vi "PathfindInner.vi"(2 "Moves Left":dbl=3.0, 3 "Pathfinding Settings":T3={"Movement Settings"={"Arrival Tolerance (m)"=0.01, "Closeness Threshold (m)"=0.5, "Pit Obstacle Radius (m)"=0.5, "Pit Locations"=[]}, "Dead Zone"=0.75, "Max Moves"=3.0, "Move Segment Length (m)"=0.02, "Path Cost Weights"={"Length Weight"=1.0, "Angle Weight"=0.0, "Angle Error Weight"=1000.0, "Angle Error Threshold"=0.314, "Per Move Penalty"=0.05, "Closeness Weight"=100.0, "Too Short Penalty"=100.0, "Too Short Threshold"=1.5}, "Desperation - Reduction Per Attempt (Ratio)"=0.9, "Desperation - Min Turning Radius (Ratio)"=0.7, "Log All Move Points"=FALSE, "Intermediate Position Grids"=[{"x1"=0.0, "x2"=1.75, "resolution"=0.15}, {"x1"=1.75, "x2"=7.38, "resolution"=0.4}]}, 4 "Turn Radius (m)":dbl=1.75, 5 "Specified End Angle":bool, 6 "Destination":cluster{"x":dbl, "y":dbl, "angle":dbl}={"x"=0.8413200000000001, "y"=0.7749, "angle"=0.0}, 7 "Start Vector":cluster{"x":dbl, "y":dbl, "angle":dbl}={"x"=5.65308, "y"=2.45016, "angle"=3.3379421944391554}) -> (0 "Total Paths Checked":dbl, 1 "Paths To Dest":T1[](array[typedef]))   [LabVIEW 2015, in "Navigation2017.lvlib" / "Navigation2017-SubVIs.lvlib"]
uses:
  Navigation2017-SubVIs.lvlib
  PathfindingSettings.ctl
  MovementSettings.ctl
  PathCostWeights.ctl
  IntermediatePositionGrids.ctl
  Path.ctl
  Move.ctl
  <vilib>/Analysis/coordinate.llb/Absolute Angle Difference (scalar).vi
  <vilib>/Analysis/coordinate.llb/Wrap Angle (scalar).vi
  <vilib>/Analysis/coordinate.llb/Set Angle Unit.vi
  Navigation2017.lvlib
  Navigation2017-util.lvlib
  <vilib>/Analysis/NI_AAL_Angle.lvlib
panel:
  # "OUTPUTS"
  # "INPUTS"
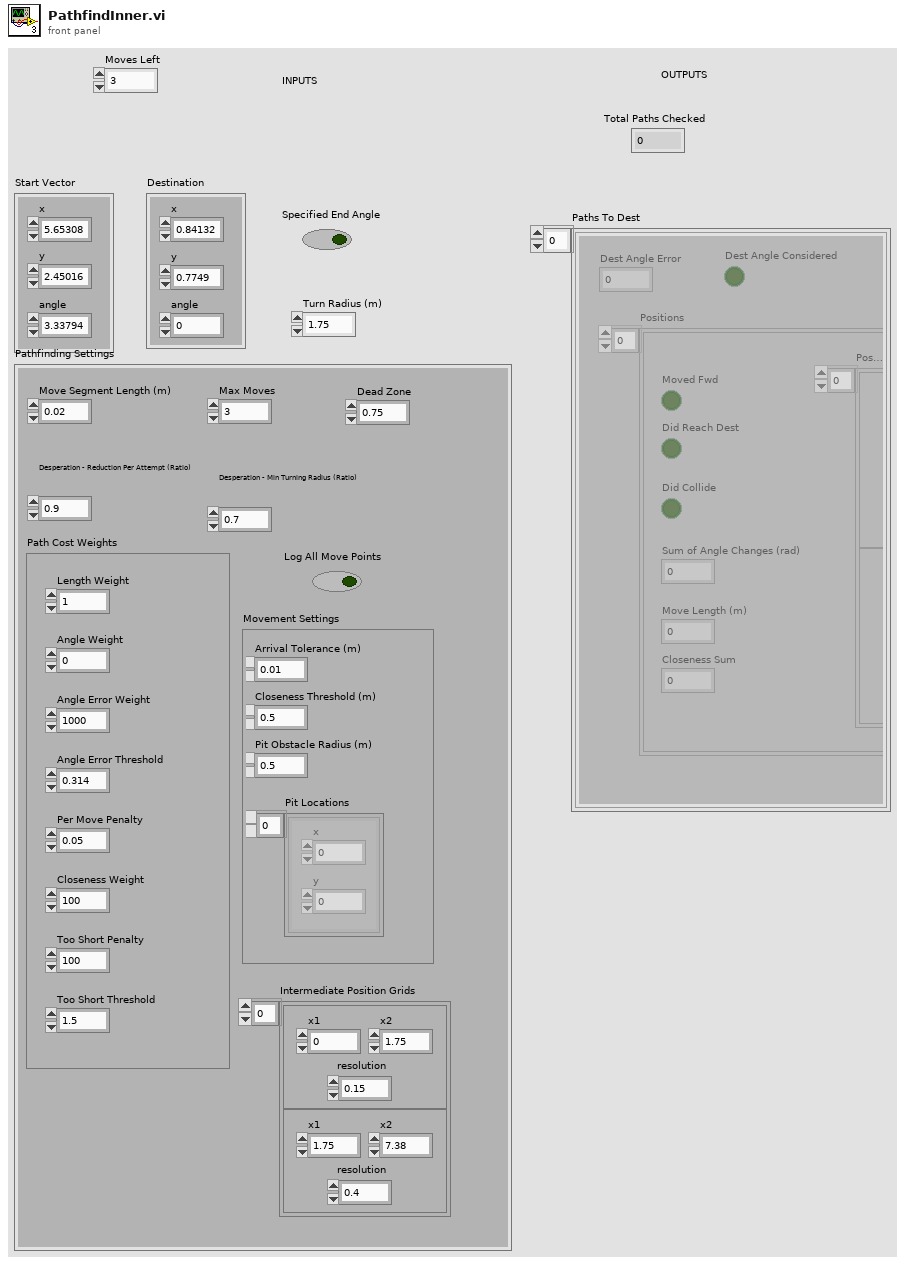
[diagram p1: front panel]
types:
  T1 = typedef "Navigation2017.lvlib/Path.ctl" = cluster{"Dest Angle Error":dbl, "Dest Angle Considered":bool, "Positions":T2[]}
  T2 = typedef "Navigation2017.lvlib/Move.ctl" = cluster{"Did Reach Dest":bool, "Did Collide":bool, "Sum of Angle Changes (rad)":dbl, "Move Length (m)":dbl, "Closeness Sum":dbl, "Positions Along Move":cluster{"x":dbl, "y":dbl, "angle":dbl}[], "Moved Fwd":bool}
  T3 = typedef "Navigation2017.lvlib/PathfindingSettings.ctl" = cluster{"Movement Settings":T4, "Dead Zone":dbl, "Max Moves":dbl, "Move Segment Length (m)":dbl, "Path Cost Weights":T5, "Desperation - Reduction Per Attempt (Ratio)":dbl, "Desperation - Min Turning Radius (Ratio)":dbl, "Log All Move Points":bool, "Intermediate Position Grids":T6}
  T4 = typedef "Navigation2017.lvlib/MovementSettings.ctl" = cluster{"Arrival Tolerance (m)":dbl, "Closeness Threshold (m)":dbl, "Pit Obstacle Radius (m)":dbl, "Pit Locations":cluster{"x":dbl, "y":dbl}[]}
  T5 = typedef "Navigation2017.lvlib/PathCostWeights.ctl" = cluster{"Length Weight":dbl, "Angle Weight":dbl, "Angle Error Weight":dbl, "Angle Error Threshold":dbl, "Per Move Penalty":dbl, "Closeness Weight":dbl, "Too Short Penalty":dbl, "Too Short Threshold":dbl}
  T6 = typedef "Navigation2017.lvlib/IntermediatePositionGrids.ctl" = cluster{"x1":dbl, "x2":dbl, "resolution":dbl}[]
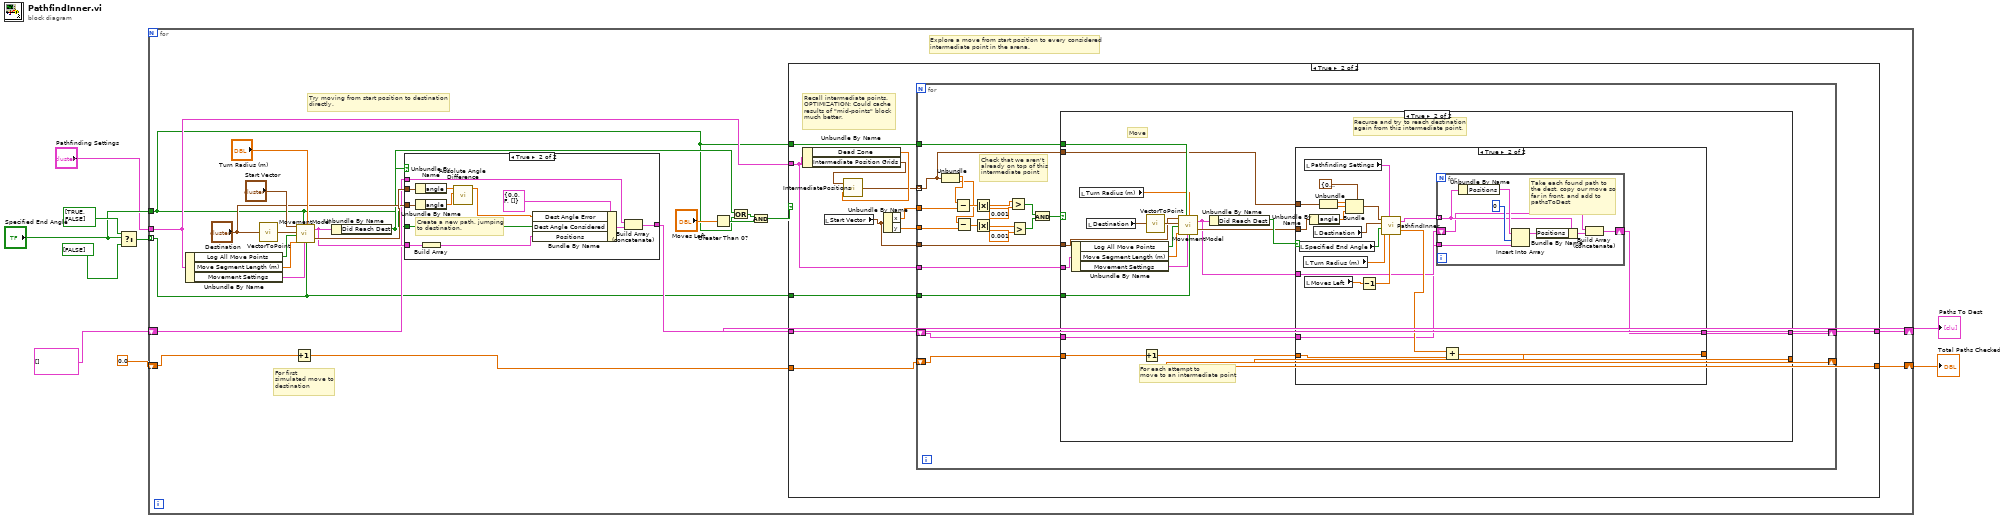
[diagram p0: block diagram]
diagram:
  n1 = Select(t=bool[] [TRUE, FALSE], s="Specified End Angle", f=bool[] [FALSE]) -> (s? t:f=w7:bool[])
  n2 = for {
    tunnel: w7 -> [w11] mode=indexing
    tunnel: "Specified End Angle" -> [w12]
    tunnel: "Pathfinding Settings" -> [w13]
    shift-right: [w20] -> w1
    shift-left: 0.0 -> [w26]
    shift-right: [w10] -> w2
    shift-left: T1[] [] -> [w22]
    # "Explore a move from start position to every considered\nintermediate point in the arena."
    # "Try moving from start position to destination\ndirectly."
    # "For first\nsimulated move to\ndestination"
    n3 = Unbundle By Name(w13) -> ("Log All Move Points"=w29:bool, "Move Segment Length (m)"=w28:dbl, "Movement Settings"=w27:T4)
    n4 = call "VectorToPoint.vi"("Vector"="Destination") -> ("Point"=w30:cluster{"x":dbl, "y":dbl})
    n5 = Increment(x=w26) -> (x+1=w19:dbl)
    n6 = call "MovementModel.vi"("Start Vector"="Start Vector", "Destination"=w30, "Log All Points"=w29, "Segment Length (m)"=w28, "Do Force Direction"=w12, "Movement Settings"=w27, "Turn Radius (m)"="Turn Radius (m)", "Force Direction Forward (If Forcing)"=w11) -> ("Move"=w23:T2, "Final Position"=w25:cluster{"x":dbl, "y":dbl, "angle":dbl})  [unwired: 10 in]
    n7 = Unbundle By Name(w23) -> ("Did Reach Dest"=w18:bool)
    n8 = case shown="True" w18 {
      tunnel: w12 -> [_ w132]
      tunnel: w25 -> [_ w130]
      tunnel: "Destination" -> [_ w129]
      tunnel: w23 -> [_ w125]
      tunnel: [w121 w122] -> w21
      tunnel: w22 -> [w121 w124]
      frame False {
      }
      frame True {
        # "Create a new path, jumping\nto destination."
        n9 = Unbundle By Name(w130) -> ("angle"=w127:dbl)
        n10 = Unbundle By Name(w129) -> ("angle"=w128:dbl)
        n11 = Build Array(w125) -> (w126:T2[])
        n12 = call-poly <vilib>:"Absolute Angle Difference.vi"("angle 2"=w128, "angle 1"=w127) -> ("absolute angle difference"=w131:dbl)  [unwired: 8 in, 1 out]
        n13 = Bundle By Name(cluster=T1 {"Dest Angle Error"=0.0, "Dest Angle Considered"=FALSE, "Positions"=[]} ("Best Path"), "Dest Angle Error"=w131, "Dest Angle Considered"=w132, "Positions"=w126) -> (w123:T1)
        n14 = Build Array (concatenate)(w124, w123) -> (w122:T1[])
      }
    }
    n15 = Greater Than 0?(x="Moves Left") -> (x > 0?=w15:bool)
    n16 = Or(x=w18, y=w12) -> (x .or. y?=w17:bool)
    n17 = And(x=w17, y=w15) -> (x .and. y?=w16:bool)
    n18 = case shown="True" w16 {
      tunnel: [w34 w36] -> w10
      tunnel: w21 -> [w34 w35]
      tunnel: [w33 w43] -> w20
      tunnel: w19 -> [w33 w44]
      tunnel: w13 -> [_ w39]
      tunnel: w12 -> [_ w38]
      tunnel: w11 -> [_ w37]
      frame False {
      }
      frame True {
        # "Recall intermediate points.\nOPTIMIZATION: Could cache\nresults of \"mid-points\" block\nmuch better."
        n19 = Unbundle By Name(w39) -> ("Dead Zone"=w46:dbl, "Intermediate Position Grids"=w47:T6)
        n20 = local read "Start Vector"() -> (w40:cluster{"x":dbl, "y":dbl, "angle":dbl})
        n21 = call "IntermediatePositions.vi"("Dead Zone"=w46, "Position Grids"=w47) -> ("Positions"=w45:cluster{dbl, dbl}[])
        n22 = Unbundle By Name(w40) -> ("x"=w42:dbl, "y"=w41:dbl)
        n23 = for {
          tunnel: w45 -> [w50] mode=indexing
          shift-right: [w52] -> w43
          shift-left: w44 -> [w51]
          tunnel: w42 -> [w61]
          tunnel: w41 -> [w60]
          tunnel: w40 -> [w56]
          tunnel: w39 -> [w55]
          tunnel: w38 -> [w54]
          tunnel: w37 -> [w53]
          shift-right: [w48] -> w36
          shift-left: w35 -> [w49]
          # "Check that we aren't \nalready on top of this\nintermediate point"
          n24 = Unbundle(w50) -> (w63:dbl, w62:dbl)
          n25 = Subtract(x=w63, y=w61) -> (x-y=w65:dbl)
          n26 = Subtract(x=w62, y=w60) -> (x-y=w64:dbl)
          n27 = Absolute Value(x=w65) -> (abs(x)=w69:dbl)
          n28 = Absolute Value(x=w64) -> (abs(x)=w68:dbl)
          n29 = Greater?(x=w69, y=0.001) -> (0:w59:bool)
          n30 = Greater?(x=w68, y=0.001) -> (0:w58:bool)
          n31 = And(x=w59, y=w58) -> (x .and. y?=w57:bool)
          n32 = case shown="True" w57 {
            tunnel: w56 -> [_ w88]
            tunnel: w55 -> [_ w87]
            tunnel: w54 -> [_ w84]
            tunnel: w53 -> [_ w81]
            tunnel: [w71 w77] -> w52
            tunnel: w51 -> [w71 w80]
            tunnel: w50 -> [_ w76]
            tunnel: w49 -> [w70 w73]
            tunnel: [w70 w72] -> w48
            frame False {
            }
            frame True {
              # "For each attempt to\nmove to an intermediate point"
              # "Recurse and try to reach destination\nagain from this intermediate point."
              # "Move"
              n33 = Unbundle By Name(w87) -> ("Log All Move Points"=w86:bool, "Move Segment Length (m)"=w85:dbl, "Movement Settings"=w82:T4)
              n34 = local read "Turn Radius (m)"() -> (w83:dbl)
              n35 = local read "Destination"() -> (w90:cluster{"x":dbl, "y":dbl, "angle":dbl})
              n36 = Increment(x=w80) -> (x+1=w78:dbl)
              n37 = call "VectorToPoint.vi"("Vector"=w90) -> ("Point"=w89:cluster{"x":dbl, "y":dbl})
              n38 = call "MovementModel.vi"("Start Vector"=w88, "Destination"=w89, "Log All Points"=w86, "Segment Length (m)"=w85, "Do Force Direction"=w84, "Movement Settings"=w82, "Turn Radius (m)"=w83, "Force Direction Forward (If Forcing)"=w81) -> ("Move"=w74:T2, "Final Position"=w75:cluster{"x":dbl, "y":dbl, "angle":dbl})  [unwired: 10 in]
              n39 = Unbundle By Name(w74) -> ("Did Reach Dest"=w79:bool)
              n40 = case shown="True" w79 {
                tunnel: w78 -> [w92 w111]
                tunnel: [w92 w110] -> w77
                tunnel: w76 -> [_ w108]
                tunnel: w75 -> [_ w105]
                tunnel: w74 -> [_ w95]
                tunnel: w73 -> [w91 w94]
                tunnel: [w91 w93] -> w72
                frame False {
                }
                frame True {
                  n41 = local read "Specified End Angle"() -> (w101:bool)
                  n42 = local read "Turn Radius (m)"() -> (w100:dbl)
                  n43 = local read "Pathfinding Settings"() -> (w97:T3)
                  n44 = local read "Moves Left"() -> (w99:dbl)
                  n45 = Unbundle By Name(w105) -> ("angle"=w104:dbl)
                  n46 = local read "Destination"() -> (w102:cluster{"x":dbl, "y":dbl, "angle":dbl})
                  n47 = Unbundle(w108) -> (w107:dbl, w106:dbl)
                  n48 = Bundle(cluster=cluster{dbl, dbl, dbl} {0.0, 0.0, 0.0}, w107, w106, w104) -> (w103:cluster{dbl, dbl, dbl})
                  n49 = Decrement(x=w99) -> (x-1=w98:dbl)
                  n50 = call "PathfindInner.vi"("Moves Left"=w98, "Pathfinding Settings"=w97, "Turn Radius (m)"=w100, "Specified End Angle"=w101, "Destination"=w102, "Start Vector"=w103) -> ("Total Paths Checked"=w112:dbl, "Paths To Dest"=w96:T1[])
                  n51 = for {
                    tunnel: w96 -> [w116] mode=indexing
                    tunnel: w95 -> [w118]
                    shift-right: [w114] -> w93
                    shift-left: w94 -> [w115]
                    # "Take each found path to\nthe dest, copy our move so\nfar in front, and add to\npathsToDest"
                    n52 = Unbundle By Name(w116) -> ("Positions"=w119:T2[])
                    n53 = Insert Into Array(array=w119, index=0, new element=w118) -> (w117:T2[])
                    n54 = Bundle By Name(cluster=w116, "Positions"=w117) -> (w113:T1)
                    n55 = Build Array (concatenate)(w115, w113) -> (w114:T1[])
                  }
                  n56 = Add(x=w112, y=w111) -> (x+y=w110:dbl)
                }
              }
            }
          }
        }
      }
    }
  }
  "Total Paths Checked" <- w1
  "Paths To Dest" <- w2
